vi "FinalizeHWI.vi"(8 "error in (no error)":errorcluster, 10 "Master Device in":refnum<class "Master Device.lvclass">, 11 "Pulseblaster in":refnum<class "Pulseblaster.lvclass">) -> (0 "error out":errorcluster, 2 "Master Device out":refnum<class "Master Device.lvclass">, 3 "Pulseblaster out":refnum<class "Pulseblaster.lvclass">)   [LabVIEW 2013, in "Pulseblaster.lvclass"]
uses:
  Pulseblaster.lvclass
  Master Device/Master Device.lvclass
  Pulseblaster.lvclass/Pulseblaster.ctl
  Utils_devs/PB_HWI/PulseBlaster.lvlib
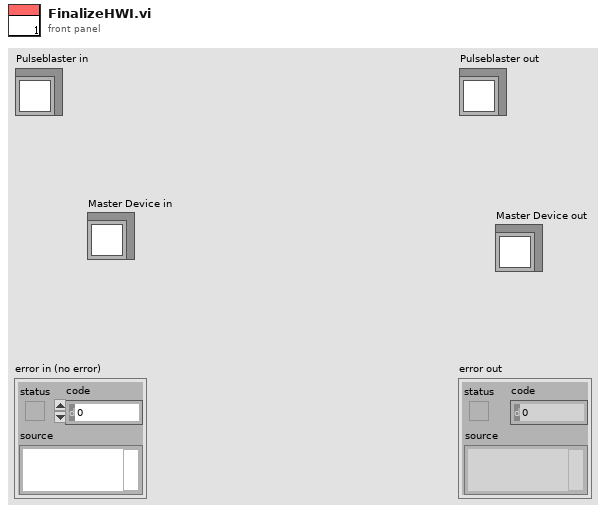
[diagram p1: front panel]
types:
  T1 = cluster{"Output Bits":u32, "Data Field":u32, "OP Code":u8, "Delay Count":u32}[]
  T2 = typedef "SlaveInfo.ctl" = cluster{"Triggering":bool[][], "Ramp Info":T3[], "Line Inversion":bool[], "Slaved Digital Channels":cluster{"Master Channel Number":i32, "Output States":bool[]}[]}
  T3 = typedef "RampInfo.ctl" = cluster{"Table Ramp Index":i32, "Ramp Time":dbl, "Number of Steps":i32, "Instruction Array Index":i32}
  T4 = cluster{"Output Bits":u32, "Data Field":u32, "OP Code":u8, "Delay Count":u64}[]
  T5 = cluster{"External MemorySize":u16, "Internal Memory Size":u16, "Overhead Ticks":u8, "Min Delay Loops":u8, "Loop Count Correction":u8, "Long Delay Loop Count Correction":u8, "Min Instruction Ticks":u8, "Long Delay Ticks":u64, "Clock Period (s)":dbl, "Overhead Time (s)":dbl, "Min Instruction Cycle Time (s)":dbl, "Long Delay Time (s) ":dbl}
  T6 = cluster{"Output Bits":u32, "Data Field":u32, "OP Code":u8, "Delay Count":u64}
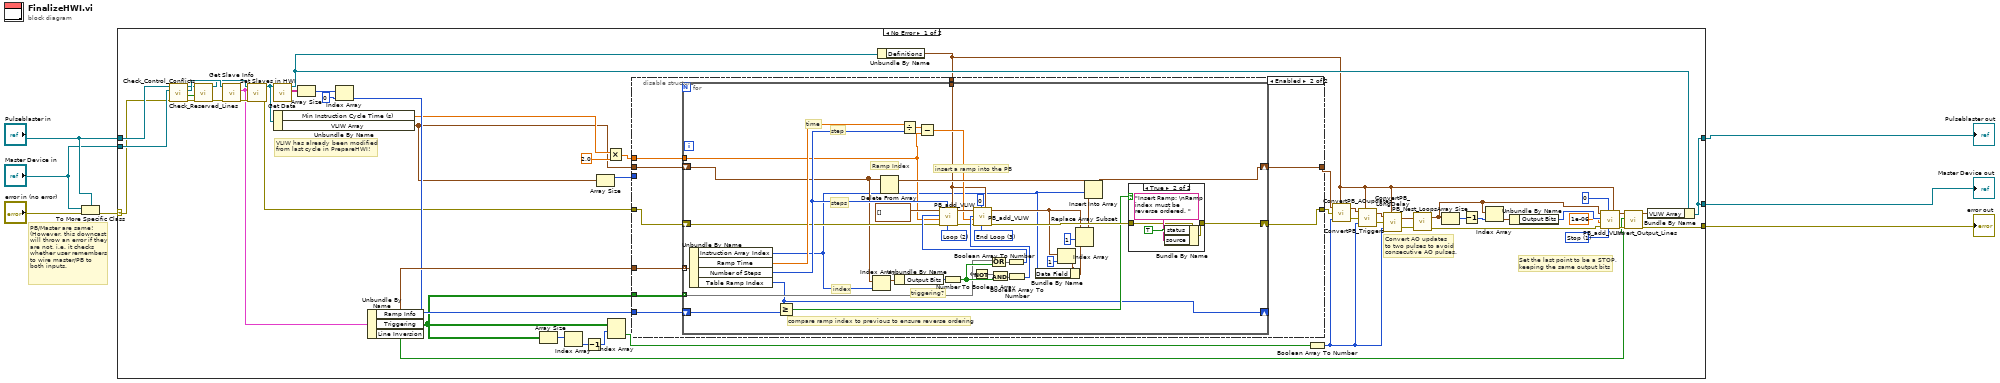
[diagram p0: block diagram]
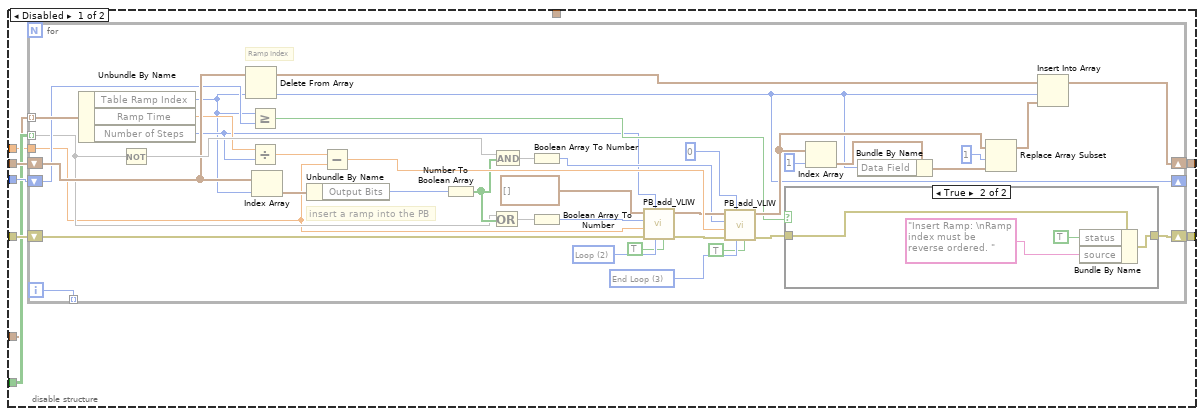
[diagram p2: hidden frame]
diagram:
  # "PB/Master are same!\n(However, this downcast\nwill throw an error if they\nare not, i.e. it checks\nwhether user remembers\nto wire master/PB to\nboth inputs."
  n1 = To More Specific Class(target class="Pulseblaster in", reference="Master Device in", error in="error in (no error)") -> (error out=w2:errorcluster)  [unwired: 1 out]
  n2 = case shown="No Error" w2 {
    selector: w2 -> [w18 w167]
    tunnel: [w21 w167] -> w7
    tunnel: [w35 w168] -> w6
    tunnel: [w35 w166] -> w5
    tunnel: "Pulseblaster in" -> [w19 w168]
    tunnel: "Master Device in" -> [w20 w166]
    frame No Error {
      w51 = u8 1 items=["Continue", "Stop", "Loop", "End Loop", "Jump", "Return", "Go To", "Long Delay"] ("OP code")
      # "VLIW has already been modified \nfrom last cycle in PrepareHWI!"
      # "Convert AO updates\nto two pulses to avoid\nconsecutive AO pulses."
      # "Set the last point to be a STOP,\nkeeping the same output bits"
      n3 = call-dynamic "Check_Control_Conflicts.vi"("error in (no error)"=w18, "Master Device in"=w20, "Device in"=w19) -> ("error out"=w15:errorcluster, "Controlled Channels"=w13:bool[], "Master Device out"=w17:refnum<class "Master Device.lvclass">, "Device out"=w14:refnum<class "Pulseblaster.lvclass">)  [unwired: 5 in]
      n4 = call-dynamic "Check_Reserved_Lines.vi"("error in (no error)"=w15, "Controlled Channels"=w13, "Pulseblaster in"=w14) -> ("error out"=w16:errorcluster, "Pulseblaster out"=w10:refnum<class "Pulseblaster.lvclass">)  [unwired: 7 in]
      n5 = call-dynamic "Get Slave Info.vi"("error in (no error)"=w16, "Master Device in"=w17) -> ("error out"=w12:errorcluster, "Slave Info"=w11:T2)  [unwired: 7 in, 1 out]
      n6 = call-dynamic "Set Slaves in HWI.vi"("error in (no error)"=w12, "Slave Info"=w11, "Pulseblaster in"=w10) -> ("error out"=w8:errorcluster, "Pulseblaster out"=w9:refnum<class "Pulseblaster.lvclass">)  [unwired: 7 in]
      n7 = call-dynamic "Get Data.vi"("Device in"=w9) -> ("Table Indicator"=w39:string[][], "Device out"=w34:refnum<class "Pulseblaster.lvclass">)  [unwired: 7 in, 1 out]
      n8 = Unbundle By Name(w9) -> ("Min Instruction Cycle Time (s)"=w28:dbl, "VLIW Array"=w27:T4)
      n9 = Array Size(array=w39) -> (size(s)=w38:i32[])
      n10 = Index Array(array=w38, index=0) -> (element=w36:i32)
      n11 = Unbundle By Name(w11) -> ("Ramp Info"=w45:T3[], "Triggering"=w26:bool[][], "Line Inversion"=w22:bool[])
      n12 = Array Size(array=w26) -> (size(s)=w42:i32[])
      n13 = Index Array(array=w42) -> (element=w40:i32)  [unwired: 1 in]
      n14 = Decrement(x=w40) -> (x-1=w41:i32)
      n15 = Array Size(array=w27) -> (size(s)=w61:i32)
      n16 = Multiply(x=w28, y=2.0) -> (x*y=w43:dbl)
      n17 = Index Array(array=w26, index (row)=w41) -> (element=w46:bool[])  [unwired: 1 in]
      n18 = Unbundle By Name(w34) -> ("Definitions"=w33:T5)
      n19 = disable-structure shown="Enabled" {
        disable-tunnel: w61 -> [w69 _]
        disable-tunnel: w27 -> [w68 w120]
        disable-tunnel: [w67 w117] -> w49
        disable-tunnel: [w66 w118] -> w48
        disable-tunnel: w8 -> [w65 w121]
        disable-tunnel: w26 -> [w64 w122]
        disable-tunnel: w45 -> [w63 w116]
        disable-tunnel: w43 -> [w62 w119]
        disable-tunnel: w36 -> [_ w115]
        disable-tunnel: w33 -> [_ w114]
        frame Disabled {
          n20 = for {
            tunnel: w63 -> [w79] mode=indexing
            shift-right: [w82] -> w67
            shift-left: w65 -> [w83]
            shift-right: [w80] -> w66
            shift-left: w68 -> [w81]
            shift-right: [w73] -> _
            shift-left: w69 -> [w77]
            tunnel: w62 -> [w74]
            tunnel: w64 -> [w76] mode=indexing
            tunnel: [w72] -> _ mode=indexing
            i -> [w72]
            w101 = u8 3 items=["Continue", "Stop", "Loop", "End Loop", "Jump", "Return", "Go To", "Long Delay"] ("OP code")
            w104 = u8 2 items=["Continue", "Stop", "Loop", "End Loop", "Jump", "Return", "Go To", "Long Delay"] ("OP code")
            # "insert a ramp into the PB"
            # "Ramp Index"
            n21 = Unbundle By Name(w79) -> ("Table Ramp Index"=w73:i32, "Ramp Time"=w78:dbl, "Number of Steps"=w75:i32)
            n22 = Not(x=w76) -> (.not. x?=w86:bool[])
            n23 = Delete From Array(array=w81, index=w73) -> (array with subset deleted=w90:T4)  [unwired: 1 in, 1 out]
            n24 = Greater Or Equal?(x=w73, y=w77) -> (x >= y?=w85:bool)
            n25 = Divide(x=w78, y=w75) -> (x/y=w108:dbl)
            n26 = Index Array(array=w81, index=w73) -> (element=w106:T6)
            n27 = Unbundle By Name(w106) -> ("Output Bits"=w91:u32)
            n28 = Subtract(x=w108, y=w74) -> (x-y=w107:dbl)
            n29 = Number To Boolean Array(number=w91) -> (Boolean array=w87:bool[])
            n30 = Or(x=w76, y=w87) -> (x .or. y?=w89:bool[])
            n31 = And(x=w86, y=w87) -> (x .and. y?=w88:bool[])
            n32 = Boolean Array To Number(Boolean array=w88) -> (number=w99:u32)
            n33 = Boolean Array To Number(Boolean array=w89) -> (number=w105:u32)
            n34 = call "PB_add_VLIW.vi"("Use Global (F)?"=TRUE, "OP code"=w104, "Data Field"=w75, "error in (no error)"=w83, "Delay"=w74, "Digital Bits"=w105, "VLIW Array In"=T1 []) -> ("error out"=w102:errorcluster, "VLIW Array Out"=w103:T4)  [unwired: 2 in, 1 out]
            n35 = call "PB_add_VLIW.vi"("Use Global (F)?"=TRUE, "OP code"=w101, "Data Field"=u32 0, "error in (no error)"=w102, "Delay"=w107, "Digital Bits"=w99, "VLIW Array In"=w103) -> ("error out"=w84:errorcluster, "VLIW Array Out"=w92:T4)  [unwired: 2 in, 1 out]
            n36 = case shown="True" w85 {
              tunnel: [w109 w111] -> w82
              tunnel: w84 -> [w109 w110]
              frame False {
              }
              frame True {
                n37 = Bundle By Name(cluster=w110, "status"=TRUE, "source"="Insert Ramp: \nRamp index must be reverse ordered. ") -> (w111:errorcluster)
              }
            }
            n38 = Index Array(array=w92, index=1 ("Index")) -> (element=w96:T6)
            n39 = Bundle By Name(cluster=w96, "Data Field"=w73) -> (w95:T6)
            n40 = Replace Array Subset(array=w92, new element=w95, index=1) -> (w93:T4)
            n41 = Insert Into Array(array=w90, index=w73, new element=w93) -> (w80:T4)
          }
        }
        frame Enabled {
          n42 = for {
            tunnel: w116 -> [w135] mode=indexing
            tunnel: w122 -> [w132] mode=indexing
            shift-right: [w130] -> w117
            shift-left: w121 -> [w131]
            shift-right: [w128] -> w118
            shift-left: w120 -> [w129]
            shift-right: [w125] -> _
            shift-left: w115 -> [w127]
            tunnel: w119 -> [w126]
            tunnel: w114 -> [w124]
            w143 = u8 3 items=["Continue", "Stop", "Loop", "End Loop", "Jump", "Return", "Go To", "Long Delay"] ("OP code")
            w140 = u8 2 items=["Continue", "Stop", "Loop", "End Loop", "Jump", "Return", "Go To", "Long Delay"] ("OP code")
            # "triggering?"
            # "compare ramp index to previous to ensure reverse ordering"
            # "steps"
            # "step"
            # "time"
            # "index"
            # "insert a ramp into the PB"
            # "Ramp Index"
            n43 = Unbundle By Name(w135) -> ("Instruction Array Index"=w123:i32, "Ramp Time"=w134:dbl, "Number of Steps"=w133:i32, "Table Ramp Index"=w125:i32)
            n44 = Greater Or Equal?(x=w125, y=w127) -> (x >= y?=w159:bool)
            n45 = Index Array(array=w129, index=w123) -> (element=w138:T6)
            n46 = Delete From Array(array=w129, index=w123) -> (array with subset deleted=w154:T4)  [unwired: 1 in, 1 out]
            n47 = Unbundle By Name(w138) -> ("Output Bits"=w153:u32)
            n48 = Divide(x=w134, y=w133) -> (x/y=w136:dbl)
            n49 = Subtract(x=w136, y=w126) -> (x-y=w137:dbl)
            n50 = Number To Boolean Array(number=w153) -> (Boolean array=w157:bool[])
            n51 = Not(x=w132) -> (.not. x?=w158:bool[])
            n52 = Or(x=w132, y=w157) -> (x .or. y?=w155:bool[])
            n53 = And(x=w158, y=w157) -> (x .and. y?=w156:bool[])
            n54 = Boolean Array To Number(Boolean array=w155) -> (number=w139:u32)
            n55 = call "PB_add_VLIW.vi"("Definitions"=w124, "OP code"=w140, "Data Field"=w133, "error in (no error)"=w131, "Delay"=w126, "Digital Bits"=w139, "VLIW Array In"=T1 []) -> ("error out"=w142:errorcluster, "VLIW Array Out"=w141:T4)  [unwired: 2 in, 1 out]
            n56 = Boolean Array To Number(Boolean array=w156) -> (number=w145:u32)
            n57 = call "PB_add_VLIW.vi"("Definitions"=w124, "OP code"=w143, "Data Field"=u32 0, "error in (no error)"=w142, "Delay"=w137, "Digital Bits"=w145, "VLIW Array In"=w141) -> ("error out"=w160:errorcluster, "VLIW Array Out"=w152:T4)  [unwired: 2 in, 1 out]
            n58 = Index Array(array=w152, index=1 ("Index")) -> (element=w148:T6)
            n59 = Bundle By Name(cluster=w148, "Data Field"=w123) -> (w149:T6)
            n60 = Replace Array Subset(array=w152, new element=w149, index=1) -> (w151:T4)
            n61 = Insert Into Array(array=w154, index=w123, new element=w151) -> (w128:T4)
            n62 = case shown="True" w159 {
              tunnel: [w161 w163] -> w130
              tunnel: w160 -> [w161 w162]
              frame False {
              }
              frame True {
                n63 = Bundle By Name(cluster=w162, "status"=TRUE, "source"="Insert Ramp: \nRamp index must be reverse ordered. ") -> (w163:errorcluster)
              }
            }
          }
        }
      }
      n64 = Boolean Array To Number(Boolean array=w46) -> (number=w47:u32)
      n65 = call "ConvertPB_AOupdates.vi"("PB VLIW Array in"=w48, "Definitions"=w33, "error in (no error)"=w49, "Full trigger mask"=w47) -> ("PB VLIW Array out"=w57:T4, "error out"=w58:errorcluster)  [unwired: 1 in]
      n66 = call "ConvertPB_Triggers.vi"("PB VLIW Array in"=w57, "Definitions"=w33, "error in (no error)"=w58, "Full trigger mask"=w47) -> ("PB VLIW Array out"=w59:T4, "error out"=w60:errorcluster)  [unwired: 1 in]
      n67 = call "ConvertPB_LongDelay.vi"("PB VLIW Array in"=w59, "Definitions"=w33, "error in (no error)"=w60, "Full trigger mask"=w47) -> ("PB VLIW Array out"=w31:T4, "error out"=w32:errorcluster)  [unwired: 1 in]
      n68 = call "PB_Nest_Loops.vi"("error in (no error)"=w32, "PB VLIW Array in"=w31) -> ("error out"=w29:errorcluster, "PB VLIW Array out"=w30:T4)
      n69 = Array Size(array=w30) -> (size(s)=w55:i32)
      n70 = Decrement(x=w55) -> (x-1=w54:i32)
      n71 = Index Array(array=w30, index=w54) -> (element=w53:T6)
      n72 = Unbundle By Name(w53) -> ("Output Bits"=w56:u32)
      n73 = call "PB_add_VLIW.vi"("Definitions"=w33, "OP code"=w51, "Data Field"=0, "error in (no error)"=w29, "Delay"=1e-06, "Digital Bits"=w56, "VLIW Array In"=w30) -> ("error out"=w25:errorcluster, "VLIW Array Out"=w24:T4)  [unwired: 2 in, 1 out]
      n74 = call "Invert_Output_Lines.vi"("Error In"=w25, "Line Inversion Array"=w22, "VLIW Array In"=w24) -> ("Error Out"=w21:errorcluster, "VLIW Array Out"=w23:T4)  [unwired: 7 in]
      n75 = Bundle By Name(cluster=w34, "VLIW Array"=w23) -> (w35:refnum<class "Pulseblaster.lvclass">)
    }
    frame Error {
    }
  }
  "error out" <- w7
  "Pulseblaster out" <- w6
  "Master Device out" <- w5
